vi "Update WayPt Angles.vi"(6 "Min R":dbl, 8 "Blends In":T1[](array[typedef]), 9 "Index":i32, 10 "Waypoints in":cluster{"x":dbl, "y":dbl, "th":dbl}[](array[cluster]), 11 "th":dbl) -> (1 "Blends Out":T1[](array[typedef]), 3 "Waypoints out":cluster{"x":dbl, "y":dbl, "th":dbl}[](array[cluster]))   [LabVIEW 2020]
uses:
  BlendType.ctl
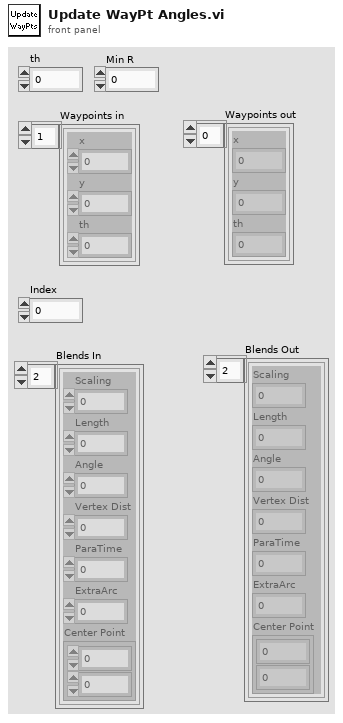
[diagram p1: front panel]
types:
  T1 = typedef "BlendType.ctl" = cluster{"Scaling":dbl, "Length":dbl, "Angle":dbl, "Vertex Dist":dbl, "ParaTime":dbl, "ExtraArc":dbl, "Center Point":cluster{dbl, dbl}}
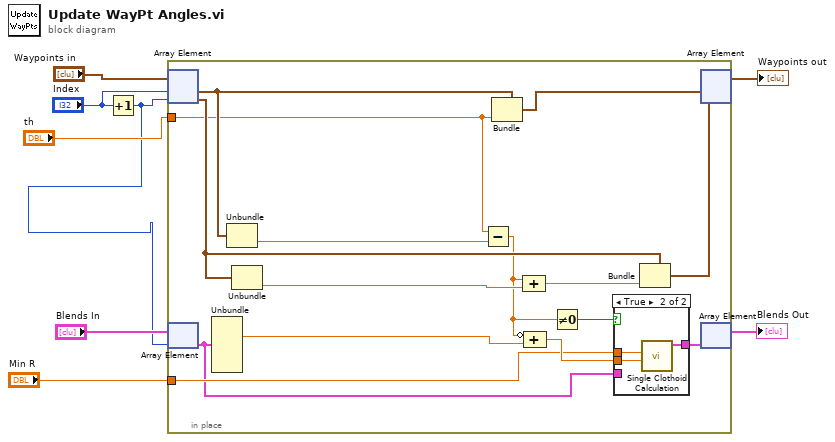
[diagram p0: block diagram]
diagram:
  n1 = Increment(x="Index") -> (x+1=w1:i32)
  n2 = in-place {
    in-place-border: "th" -> [w10]
    in-place-border: "Min R" -> [w15]
    n3 = in-place-array #1("Waypoints in", "Index", w1) -> (w19:cluster{"x":dbl, "y":dbl, "th":dbl}, w22:cluster{"x":dbl, "y":dbl, "th":dbl})
    n4 = in-place-array #2("Blends In", w1) -> (w13:T1)
    n5 = Unbundle(w13) -> ("Angle"=w17:dbl)  [unwired: 6 out]
    n6 = Unbundle(w19) -> ("th"=w9:dbl)  [unwired: 2 out]
    n7 = Unbundle(w22) -> ("th"=w20:dbl)  [unwired: 2 out]
    n8 = Subtract(x=w10, y=w9) -> (x-y=w12:dbl)
    n9 = Bundle(cluster=w19, "th"=w10) -> (w23:cluster{"x":dbl, "y":dbl, "th":dbl})  [unwired: 2 in]
    n10 = Compound Arithmetic op=ADD(w12, w20) -> (w18:dbl)
    n11 = Compound Arithmetic op=ADD(invert w12, w17) -> (w16:dbl)
    n12 = Not Equal To 0?(x=w12) -> (x != 0?=w11:bool)
    n13 = case shown="True" w11 {
      tunnel: w16 -> [_ w27]
      tunnel: w15 -> [_ w26]
      tunnel: [w24 w25] -> w14
      tunnel: w13 -> [w24 _]
      frame False {
      }
      frame True {
        n14 = call "Single Clothoid Calculation.vi"("Angle"=w27, "Min R"=w26) -> ("Zeroes out"=w25:T1)  [unwired: 9 in]
      }
    }
    n15 = Bundle(cluster=w22, "th"=w18) -> (w21:cluster{"x":dbl, "y":dbl, "th":dbl})  [unwired: 2 in]
    n16 = in-place-array #1(w23, w21) -> (→"Waypoints out":cluster{"x":dbl, "y":dbl, "th":dbl}[])  [unwired: 2 out]
    n17 = in-place-array #2(w14) -> (→"Blends Out":T1[])  [unwired: 1 out]
  }
